vi "Terminal-PressureSystemLubricateUnit-ParametersSetter.vi"(8 "error in (no error)":errorcluster caption="错误输入（无错误）", 9 "供油润滑温度T":u16, 10 "供油流量L":u16, 11 "write operation timeout (ms)":i32=5000 caption="写操作超时（5000毫秒）") -> (0 "error out":errorcluster caption="错误输出")   [LabVIEW 2014]
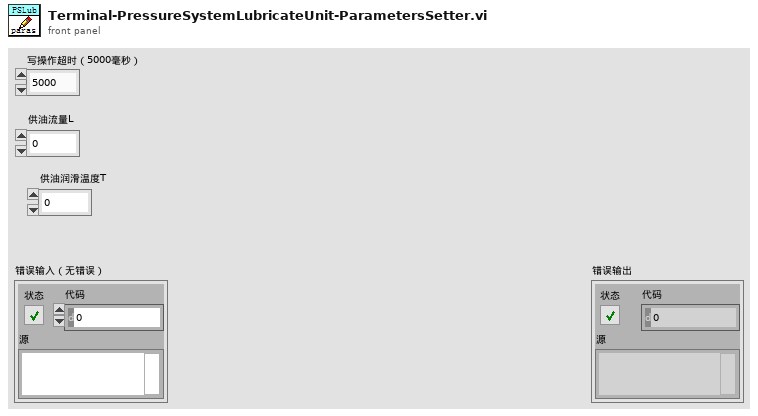
[diagram p1: front panel]
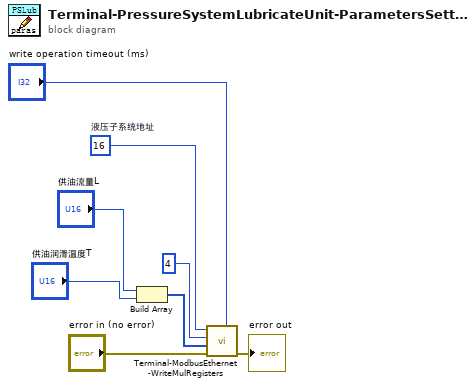
[diagram p0: block diagram]
diagram:
  w6 = u8 16  # 液压子系统地址
  n1 = Build Array("供油流量L", "供油润滑温度T") -> (w3:u16[])
  n2 = call "Terminal-ModbusEthernet-WriteMulRegisters.vi"("write operation timeout (ms)"="write operation timeout (ms)", "error in"="error in (no error)", "holding register values"=w3, "starting address"=u16 4 ("address"), "unit ID"=w6) -> ("error out"=→"error out":errorcluster)  [unwired: 6 in]
